vi "Write scale maximum.vi"(8 "error in (no error)":errorcluster, 10 "scale maximum":dbl=100.0, 11 "Y_H in":refnum<class "Y_H.lvclass">) -> (0 "error out":errorcluster, 3 "Y_H out":refnum<class "Y_H.lvclass">)   [LabVIEW 2019, in "Y_H.lvclass"]
uses:
  Y_H.lvclass
  Y_H.lvclass/Y_H.ctl
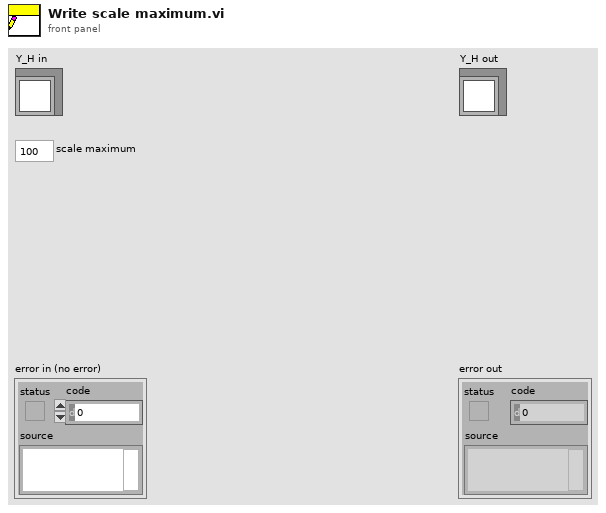
[diagram p1: front panel]
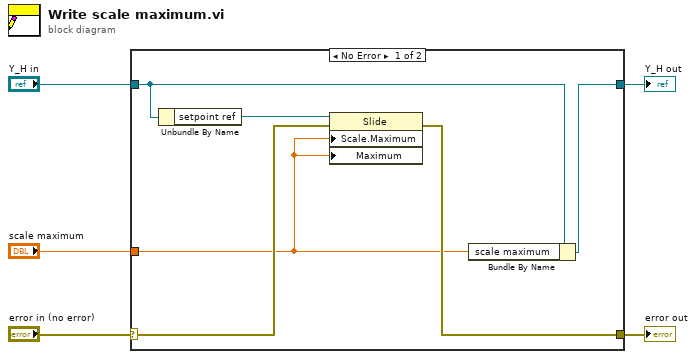
[diagram p0: block diagram]
diagram:
  n1 = case shown="No Error" "error in (no error)" {
    selector: "error in (no error)" -> [w8 w12]
    tunnel: [w7 w12] -> w4
    tunnel: [w11 w13] -> w2
    tunnel: "Y_H in" -> [w10 w13]
    tunnel: "scale maximum" -> [w6 _]
    frame No Error {
      n2 = Unbundle By Name(w10) -> ("setpoint ref"=w9:refnum<vi>)
      n3 = property on="Property Node" class="Slide"(reference=w9, error in=w8, "Scale.Maximum"=w6, "Maximum"=w6) -> (error out=w7:errorcluster)  [unwired: 1 out]
      n4 = Bundle By Name(cluster=w10, "scale maximum"=w6) -> (w11:refnum<class "Y_H.lvclass">)
    }
    frame Error {
    }
  }
  "error out" <- w4
  "Y_H out" <- w2
